vi "XLP80_CAN_VerifyEnums.vi"(8 "err in":errorcluster caption="error") -> (0 "err out":errorcluster caption="error")   [LabVIEW 2021]
uses:
  XLP80_FGlob/1886_FGlob_TDefEnumCANReadItems_Testmode_A.ctl
  XLP80_FGlob/1886_FGlob_TDefEnumCANWriteItems.ctl
  XLP80_Globals/Globals_Settings_XLP80.vi
panel:
  in  "CAN Write Items Testmode_A":T1
  in  "CAN Read Items Testmode_A":T2
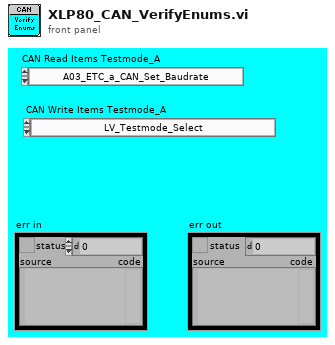
[diagram p1: front panel]
types:
  T1 = typedef "1886_FGlob_TDefEnumCANWriteItems.ctl" = enum16{"LV_Testmode_Select", "LV_A_71_Current_Out_Set", "LV_A_71_Voltage_In_Set", "LV_A_71_Voltage_Out_Set", "LV_H_51_STK_CellVoltages_Enable", "S80_BP_s_Taster_Start_Status"}
  T2 = typedef "1886_FGlob_TDefEnumCANReadItems_Testmode_A.ctl" = enum16{"A03_ETC_a_CAN_Set_Baudrate", "A03_ETC_a_CAN_Set_Broadcast", "A03_ETC_a_CAN_Set_ID_Offset", "A03_ETC_a_CAN_Set_Termination", "A03_ETC_a_CAN_Set_Timeout", "A03_ETC_a_CAN_Set_Timeout_Dur", "A03_ETC_a_Diag_Rq_Select", "A03_ETC_a_Info_Rq_Select", "A03_ETC_a_opCmd1_Error_Ack", "A03_ETC_a_opCmd1_Start_Stop", "A03_ETC_a_opCmd2", "A03_ETC_a_Param_Rq_Select", "A03_ETC_a_SP_In_Press_Enable", "A03_ETC_a_SP_In_Temp_Enable", "A03_ETC_a_SP_Inlet_Pressure", "A03_ETC_a_SP_Inlet_Temperature", "A03_ETC_a_SP_Massflow", "A03_ETC_a_SP_Massflow_Enable", "A03_ETC_a_SP_Out_Press_Enable", "A03_ETC_a_SP_Outlet_Pressure", "A03_ETC_a_Speed_Set", "A03_ETC_s_Converter_Temperature", "A03_ETC_s_Error_Code_1", "A03_ETC_s_Error_Code_2", "A03_ETC_s_HV_In_Voltage", "A03_ETC_s_Information_Code", "A03_ETC_s_LV_In_Voltage", "A03_ETC_s_Output_Power", "A03_ETC_s_Phase_Current", "A03_ETC_s_Phase_Current_Ref", "A03_ETC_s_Phase_Voltage", "A03_ETC_s_PT100_Temperature", "A03_ETC_s_Speed_Actual", "A03_ETC_s_Speed_Reference", "A03_ETC_s_Status1", "A03_ETC_s_Status2", "A03_ETC_s_THC_Temperature", "A03_ETC_s_Warning_Code", "A11_HBV_a_Mode_Set", "A11_HBV_a_Valve_Set", "A11_HBV_s_Mode_Act", "A11_HBV_s_Valve_Act", "A12_SIV_a_Mode_Set", "A12_SIV_a_Valve_Set", "A12_SIV_s_Mode_Act", "A12_SIV_s_Valve_Act", "A13_SOV_a_Mode_Set", "A13_SOV_a_Valve_Set", "A13_SOV_s_Mode_Act", "A13_SOV_s_Valve_Act", "A14_HFM_s_AirMassFlow", "A14_HFM_s_Error_MassFlow", "A14_HFM_s_Error_Pressure", "A14_HFM_s_ErrorCode", "A14_HFM_s_Humidity", "A14_HFM_s_HumidTemperature", "A14_HFM_s_Pressure", "A14_HFM_s_Temperature", "A15_SI_s_Inlet_Pressure", "A16_SI_s_Inlet_Temperature", "A17_SO_s_Outlet_Pressure", "A17_SO_s_Outlet_Temperature", "A22_HSI_s_Humidity", "A23_HSO_s_Humidity", "A56_SO_s_Temperature", "C01_RF_a_FanSpeed", "C01_RF_s_Status", "C02_CP_a_RPM", "C04_DI_s_Temperature", "C06_ET_s_CoolLevelStatus", "C07_BAT_s_BatError_DataValid", "C07_BAT_s_BatError_Intern", "C07_BAT_s_BatError_Temperature", "C07_BAT_s_BatError_Voltage", "C07_BAT_s_Battery_Voltage", "C07_BAT_s_Board_Temperature", "C07_BAT_s_CECUError_Communicat", "C07_BAT_s_CECUError_Current", "C07_BAT_s_CECUError_Intern", "C07_BAT_s_CECUError_Reserved", "C07_BAT_s_CECUError_Service", "C07_BAT_s_CECUError_Supply", "C07_BAT_s_CECUError_Temperature", "C07_BAT_s_CECUError_Voltage", "C07_BAT_s_External_Chrg_Voltage", "C07_BAT_s_External_Load_Voltage", "C07_BAT_s_Max_Cell_Temperature", "C07_BAT_s_Max_Cell_Voltage", "C07_BAT_s_Min_Cell_Temperature", "C07_BAT_s_Min_Cell_Voltage", "C07_BAT_s_PreWarning_Current_H", "C07_BAT_s_PreWarning_SOC_Low", "C07_BAT_s_PreWarning_Temperature", "C07_BAT_s_PreWarning_Voltage_HL", "C07_BAT_s_State", "C07_BAT_s_System_Current", "C08_AMB_s_Humidity_Rel", "C08_AMB_s_Humidity_Spec", "C08_AMB_s_Pressure", "C08_AMB_s_Temperature", "C54_SI_s_Temperature", "C_07_BAT_s_SoC", "C_07_BAT_s_SoH", "E71_DC4880_a_Current_In_Set", "E71_DC4880_a_Current_Out_Set", "E71_DC4880_a_Mode_Control_On", "E71_DC4880_a_Mode_Precharge_On", "E71_DC4880_a_NMT_Function", "E71_DC4880_a_NMT_Node_ID", "E71_DC4880_a_Voltage_In_Set", "E71_DC4880_a_Voltage_Out_Set", "E71_DC4880_s_Current_In_Actual", "E71_DC4880_s_Current_Out_Actual", "E71_DC4880_s_NMT_State", "E71_DC4880_s_State_Control_OK", "E71_DC4880_s_State_Control_On", "E71_DC4880_s_State_Precharge_On", "E71_DC4880_s_Temperature_1_Act", "E71_DC4880_s_Temperature_2_Act", "E71_DC4880_s_Voltage_In_Actual", "E71_DC4880_s_Voltage_Out_Actual", "E72_DC8024_s_Voltage", "E73_DC8012_s_Voltage", "E74_ISO_a_Rq_D_IMC_MANUFACT_IDX", "E74_ISO_a_Rq_D_IMC_MEAN_FACTOR", "E74_ISO_a_Rq_D_IMC_R_ISOERR_THR", "E74_ISO_a_Rq_D_IMC_R_ISOWRN_THR", "E74_ISO_a_Rq_D_IMC_SELFTEST_SCR", "E74_ISO_a_Rq_D_IMC_VERSION_IDX", "E74_ISO_a_Rq_D_VIFC_HV_REL_CHG", "E74_ISO_a_Rq_D_VIFC_HV_RELAIS", "E74_ISO_a_Rq_D_VIFC_LOCK_MODE", "E74_ISO_a_Rq_D_VIFC_LOCK_PWD", "E74_ISO_a_Rq_D_VIFC_MEAS_MODE", "E74_ISO_a_Rq_D_VIFC_RELAIS_STAT", "E74_ISO_a_Rq_D_VIFC_VERSION_IDX", "E74_ISO_s_D_IMC_HV_1", "E74_ISO_s_D_IMC_HV_2", "E74_ISO_s_D_IMC_MANUFACT_DATA", "E74_ISO_s_D_IMC_MANUFACT_INDEX", "E74_ISO_s_D_IMC_MEAN_FACTOR", "E74_ISO_s_D_IMC_R_ISO", "E74_ISO_s_D_IMC_R_ISO_BIAS", "E74_ISO_s_D_IMC_R_ISO_CNT", "E74_ISO_s_D_IMC_R_ISO_ERR_THR1", "E74_ISO_s_D_IMC_R_ISO_ERR_THR2", "E74_ISO_s_D_IMC_R_ISO_WRN_THR1", "E74_ISO_s_D_IMC_R_ISO_WRN_THR2", "E74_ISO_s_D_IMC_SELFTEST_SCR", "E74_ISO_s_D_IMC_STATUS", "E74_ISO_s_D_IMC_STATUS_EXT", "E74_ISO_s_D_IMC_TEST_CNT", "E74_ISO_s_D_IMC_VERSION_Haupt", "E74_ISO_s_D_IMC_VERSION_INDEX", "E74_ISO_s_D_IMC_VERSION_Neben", "E74_ISO_s_D_IMD_ERROR_CODE", "E74_ISO_s_D_IMD_FAILED_CMD", "E74_ISO_s_D_VIFC_HV_RELAIS", "E74_ISO_s_D_VIFC_HV_RELAIS_ACT", "E74_ISO_s_D_VIFC_HV_RELAIS_CHG", "E74_ISO_s_D_VIFC_HV_RELAIS_STAT", "E74_ISO_s_D_VIFC_IMC_ALIVE", "E74_ISO_s_D_VIFC_LOCK_MODE", "E74_ISO_s_D_VIFC_MEASURE_MODE", "E74_ISO_s_D_VIFC_STATUS", "E74_ISO_s_D_VIFC_VERSION_Haupt", "E74_ISO_s_D_VIFC_VERSION_INDEX", "E74_ISO_s_D_VIFC_VERSION_Neben", "E74_ISO_s_IMC_R_ISO", "E74_ISO_s_IMC_STATUS_ErrChassis", "E74_ISO_s_IMC_STATUS_Isofehler", "E74_ISO_s_IMC_STATUS_Isowarnung", "E74_ISO_s_IMC_STATUS_Kalib", "E74_ISO_s_IMC_STATUS_Selbsttest", "E74_ISO_s_IMC_STATUS_Syststoer", "E74_ISO_s_Rq_D_IMC_MEAN_FACTOR", "E74_ISO_s_VIFC_STATUS_IMC_Alive", "E74_ISO_s_VIFC_STATUS_IMC_St_OA", "E74_ISO_s_VIFC_STATUS_IMC_St_PC", "E74_ISO_s_VIFC_STATUS_IsoAlt", "E74_ISO_s_VIFC_STATUS_Isomess", "E74_ISO_s_VIFC_STATUS_Stoer_IMC", "E74_ISO_s_VIFC_STATUS_VIFC_Cmd", "E75_HVP_a_Relais_Set", "E76_HVM_a_Relais_Set", "E95_DC2405_s_Voltage", "H31_OTV_a_Valve_Set", "H31_OTV_s_Pressure", "H31_OTV_s_Temperature", "H36_GHU_s_Pressure_1", "H37_GHU_s_Temperature_1", "H38_HSV_a_Valve_Set", "H40_GHU_s_Pressure_2", "H41_GHU_s_Temperature_2", "H42_HRB_a_FCCU_CRC", "H42_HRB_a_FCCU_Heating_Rq", "H42_HRB_a_FCCU_Spd_Rq", "H42_HRB_a_FCCU_SQC", "H42_HRB_s_ARB_Batt_Vltg_Err", "H42_HRB_s_ARB_Batt_Voltage", "H42_HRB_s_ARB_Blocked_Err", "H42_HRB_s_ARB_BrdgDrv_Err", "H42_HRB_s_ARB_E2E_Err", "H42_HRB_s_ARB_ECU_P_out", "H42_HRB_s_ARB_ECU_Temp", "H42_HRB_s_ARB_ECU_Temp_DrCnd", "H42_HRB_s_ARB_ECU_Temp_Err", "H42_HRB_s_ARB_ErrCRC", "H42_HRB_s_ARB_ErrSQC", "H42_HRB_s_ARB_I_D_Curr", "H42_HRB_s_ARB_I_Q_Curr", "H42_HRB_s_ARB_Init_Err", "H42_HRB_s_ARB_Mtr_Temp", "H42_HRB_s_ARB_Mtr_Temp_DrCnd", "H42_HRB_s_ARB_Mtr_Temp_Err", "H42_HRB_s_ARB_MtrNTCFlr_DrCnd", "H42_HRB_s_ARB_ShortToBat_Err", "H42_HRB_s_ARB_ShortToGround_Err", "H42_HRB_s_ARB_Spd", "H42_HRB_s_ARB_SpdDiff_DrCnd", "H42_HRB_s_ARB_SpdLimitRq_Err", "H42_HRB_s_ARB_SysState", "H42_HRB_s_ARB_Torque", "H42_HRB_s_ARB_U_D_Volt", "H42_HRB_s_ARB_U_Q_Volt", "H42_HRB_s_BrdgDrv_VCC_UV_Err", "H43_HDV_a_Dosing_Valve_Set", "H45_WT_s_WaterLevelStatus", "H46_HRBo_a_Drain_Valve_Set", "H51_STK_a_AmountOfModules_1002", "H51_STK_a_CAN_TerminatRes_1002", "H51_STK_a_CellsPerModule_1002", "H51_STK_a_CellVoltage_1001", "H51_STK_a_Command_1004", "H51_STK_a_CoreData_1001", "H51_STK_a_CoreData_Freq_1002", "H51_STK_a_DataLength_1001", "H51_STK_a_DataLength_1002", "H51_STK_a_DataLength_1003", "H51_STK_a_DataLength_1004", "H51_STK_a_DataLength_1006", "H51_STK_a_DataLength_100B", "H51_STK_a_DateTime_1002", "H51_STK_a_Diff_MaxMin_limit_1002", "H51_STK_a_FCCUResponse_1006", "H51_STK_a_Firmware_1001", "H51_STK_a_ID_1003", "H51_STK_a_ID_1004", "H51_STK_a_ID_H_1001", "H51_STK_a_ID_H_1002", "H51_STK_a_ID_H_100B", "H51_STK_a_ID_L_100B", "H51_STK_a_Logdata_1001", "H51_STK_a_Lower_Limit2_1002", "H51_STK_a_MasterNo_1002", "H51_STK_a_Modul_100B", "H51_STK_a_Monitoring_Flag_1003", "H51_STK_a_PosAtStack_1002", "H51_STK_a_StackSize_1002", "H51_STK_a_Temperature_1002", "H51_STK_a_Upper_Limit1_1002", "H51_STK_a_UpperLimit2_1002", "H51_STK_s_Amount_Slave_Modu_2000", "H51_STK_s_AmountofContactFailure", "H51_STK_s_AmountOfFrames_2002", "H51_STK_s_AmountOfFrames_2003", "H51_STK_s_AmountOfFrames_2005", "H51_STK_s_AmountOfFrames_2006", "H51_STK_s_AmountOfFrames_2011", "H51_STK_s_AverageTemp_2004", "H51_STK_s_CellContactNr10_2006", "H51_STK_s_CellContactNr11_2006", "H51_STK_s_CellContactNr12_2006", "H51_STK_s_CellContactNr13_2006", "H51_STK_s_CellContactNr14_2006", "H51_STK_s_CellContactNr15_2006", "H51_STK_s_CellContactNr16_2006", "H51_STK_s_CellContactNr17_2006", "H51_STK_s_CellContactNr18_2006", "H51_STK_s_CellContactNr19_2006", "H51_STK_s_CellContactNr1_2006", "H51_STK_s_CellContactNr20_2006", "H51_STK_s_CellContactNr21_2006", "H51_STK_s_CellContactNr22_2006", "H51_STK_s_CellContactNr23_2006", "H51_STK_s_CellContactNr24_2006", "H51_STK_s_CellContactNr25_2006", "H51_STK_s_CellContactNr26_2006", "H51_STK_s_CellContactNr27_2006", "H51_STK_s_CellContactNr28_2006", "H51_STK_s_CellContactNr29_2006", "H51_STK_s_CellContactNr2_2006", "H51_STK_s_CellContactNr30_2006", "H51_STK_s_CellContactNr31_2006", "H51_STK_s_CellContactNr32_2006", "H51_STK_s_CellContactNr33_2006", "H51_STK_s_CellContactNr34_2006", "H51_STK_s_CellContactNr35_2006", "H51_STK_s_CellContactNr36_2006", "H51_STK_s_CellContactNr37_2006", "H51_STK_s_CellContactNr38_2006", "H51_STK_s_CellContactNr39_2006", "H51_STK_s_CellContactNr3_2006", "H51_STK_s_CellContactNr40_2006", "H51_STK_s_CellContactNr41_2006", "H51_STK_s_CellContactNr42_2006", "H51_STK_s_CellContactNr43_2006", "H51_STK_s_CellContactNr44_2006", "H51_STK_s_CellContactNr45_2006", "H51_STK_s_CellContactNr46_2006", "H51_STK_s_CellContactNr47_2006", "H51_STK_s_CellContactNr48_2006", "H51_STK_s_CellContactNr49_2006", "H51_STK_s_CellContactNr4_2006", "H51_STK_s_CellContactNr50_2006", "H51_STK_s_CellContactNr51_2006", "H51_STK_s_CellContactNr52_2006", "H51_STK_s_CellContactNr53_2006", "H51_STK_s_CellContactNr54_2006", "H51_STK_s_CellContactNr55_2006", "H51_STK_s_CellContactNr56_2006", "H51_STK_s_CellContactNr57_2006", "H51_STK_s_CellContactNr58_2006", "H51_STK_s_CellContactNr59_2006", "H51_STK_s_CellContactNr5_2006", "H51_STK_s_CellContactNr60_2006", "H51_STK_s_CellContactNr61_2006", "H51_STK_s_CellContactNr62_2006", "H51_STK_s_CellContactNr63_2006", "H51_STK_s_CellContactNr64_2006", "H51_STK_s_CellContactNr65_2006", "H51_STK_s_CellContactNr66_2006", "H51_STK_s_CellContactNr67_2006", "H51_STK_s_CellContactNr68_2006", "H51_STK_s_CellContactNr69_2006", "H51_STK_s_CellContactNr6_2006", "H51_STK_s_CellContactNr70_2006", "H51_STK_s_CellContactNr71_2006", "H51_STK_s_CellContactNr7_2006", "H51_STK_s_CellContactNr8_2006", "H51_STK_s_CellContactNr9_2006", "H51_STK_s_CellNo_2ndlow_2003", "H51_STK_s_CellNo_highest_2003", "H51_STK_s_CellNo_lowest_2003", "H51_STK_s_CellVolt_001_2005", "H51_STK_s_CellVolt_002_2005", "H51_STK_s_CellVolt_003_2005", "H51_STK_s_CellVolt_004_2005", "H51_STK_s_CellVolt_005_2005", "H51_STK_s_CellVolt_006_2005", "H51_STK_s_CellVolt_007_2005", "H51_STK_s_CellVolt_008_2005", "H51_STK_s_CellVolt_009_2005", "H51_STK_s_CellVolt_010_2005", "H51_STK_s_CellVolt_011_2005", "H51_STK_s_CellVolt_012_2005", "H51_STK_s_CellVolt_013_2005", "H51_STK_s_CellVolt_014_2005", "H51_STK_s_CellVolt_015_2005", "H51_STK_s_CellVolt_016_2005", "H51_STK_s_CellVolt_017_2005", "H51_STK_s_CellVolt_018_2005", "H51_STK_s_CellVolt_019_2005", "H51_STK_s_CellVolt_020_2005", "H51_STK_s_CellVolt_021_2005", "H51_STK_s_CellVolt_022_2005", "H51_STK_s_CellVolt_023_2005", "H51_STK_s_CellVolt_024_2005", "H51_STK_s_CellVolt_025_2005", "H51_STK_s_CellVolt_026_2005", "H51_STK_s_CellVolt_027_2005", "H51_STK_s_CellVolt_028_2005", "H51_STK_s_CellVolt_029_2005", "H51_STK_s_CellVolt_030_2005", "H51_STK_s_CellVolt_031_2005", "H51_STK_s_CellVolt_032_2005", "H51_STK_s_CellVolt_033_2005", "H51_STK_s_CellVolt_034_2005", "H51_STK_s_CellVolt_035_2005", "H51_STK_s_CellVolt_036_2005", "H51_STK_s_CellVolt_037_2005", "H51_STK_s_CellVolt_038_2005", "H51_STK_s_CellVolt_039_2005", "H51_STK_s_CellVolt_040_2005", "H51_STK_s_CellVolt_041_2005", "H51_STK_s_CellVolt_042_2005", "H51_STK_s_CellVolt_043_2005", "H51_STK_s_CellVolt_044_2005", "H51_STK_s_CellVolt_045_2005", "H51_STK_s_CellVolt_046_2005", "H51_STK_s_CellVolt_047_2005", "H51_STK_s_CellVolt_048_2005", "H51_STK_s_CellVolt_049_2005", "H51_STK_s_CellVolt_050_2005", "H51_STK_s_CellVolt_051_2005", "H51_STK_s_CellVolt_052_2005", "H51_STK_s_CellVolt_053_2005", "H51_STK_s_CellVolt_054_2005", "H51_STK_s_CellVolt_055_2005", "H51_STK_s_CellVolt_056_2005", "H51_STK_s_CellVolt_057_2005", "H51_STK_s_CellVolt_058_2005", "H51_STK_s_CellVolt_059_2005", "H51_STK_s_CellVolt_060_2005", "H51_STK_s_CellVolt_061_2005", "H51_STK_s_CellVolt_062_2005", "H51_STK_s_CellVolt_063_2005", "H51_STK_s_CellVolt_064_2005", "H51_STK_s_CellVolt_065_2005", "H51_STK_s_CellVolt_066_2005", "H51_STK_s_CellVolt_067_2005", "H51_STK_s_CellVolt_068_2005", "H51_STK_s_CellVolt_069_2005", "H51_STK_s_CellVolt_070_2005", "H51_STK_s_CellVolt_071_2005", "H51_STK_s_CellVolt_2ndlow_2003", "H51_STK_s_CellVolt_follow_2ndlow", "H51_STK_s_CellVolt_follow_lowest", "H51_STK_s_CellVolt_highest_2003", "H51_STK_s_CellVolt_lowest_2003", "H51_STK_s_CellVolt_prev_2ndlow", "H51_STK_s_CellVolt_prev_lowest", "H51_STK_s_CellVoltage_ui16H_2004", "H51_STK_s_CellVoltage_ui16L_2004", "H51_STK_s_Contact_Cell_10_2010", "H51_STK_s_Contact_Cell_11_2010", "H51_STK_s_Contact_Cell_12_2010", "H51_STK_s_Contact_Cell_13_2010", "H51_STK_s_Contact_Cell_14_2010", "H51_STK_s_Contact_Cell_15_2010", "H51_STK_s_Contact_Cell_16_2010", "H51_STK_s_Contact_Cell_17_2010", "H51_STK_s_Contact_Cell_18_2010", "H51_STK_s_Contact_Cell_19_2010", "H51_STK_s_Contact_Cell_1_2010", "H51_STK_s_Contact_Cell_20_2010", "H51_STK_s_Contact_Cell_21_2010", "H51_STK_s_Contact_Cell_22_2010", "H51_STK_s_Contact_Cell_23_2010", "H51_STK_s_Contact_Cell_24_2010", "H51_STK_s_Contact_Cell_25_2010", "H51_STK_s_Contact_Cell_26_2010", "H51_STK_s_Contact_Cell_27_2010", "H51_STK_s_Contact_Cell_28_2010", "H51_STK_s_Contact_Cell_29_2010", "H51_STK_s_Contact_Cell_2_2010", "H51_STK_s_Contact_Cell_30_2010", "H51_STK_s_Contact_Cell_31_2010", "H51_STK_s_Contact_Cell_32_2010", "H51_STK_s_Contact_Cell_33_2010", "H51_STK_s_Contact_Cell_34_2010", "H51_STK_s_Contact_Cell_35_2010", "H51_STK_s_Contact_Cell_36_2010", "H51_STK_s_Contact_Cell_37_2010", "H51_STK_s_Contact_Cell_38_2010", "H51_STK_s_Contact_Cell_39_2010", "H51_STK_s_Contact_Cell_3_2010", "H51_STK_s_Contact_Cell_40_2010", "H51_STK_s_Contact_Cell_41_2010", "H51_STK_s_Contact_Cell_42_2010", "H51_STK_s_Contact_Cell_43_2010", "H51_STK_s_Contact_Cell_44_2010", "H51_STK_s_Contact_Cell_45_2010", "H51_STK_s_Contact_Cell_46_2010", "H51_STK_s_Contact_Cell_47_2010", "H51_STK_s_Contact_Cell_48_2010", "H51_STK_s_Contact_Cell_49_2010", "H51_STK_s_Contact_Cell_4_2010", "H51_STK_s_Contact_Cell_50_2010", "H51_STK_s_Contact_Cell_51_2010", "H51_STK_s_Contact_Cell_52_2010", "H51_STK_s_Contact_Cell_53_2010", "H51_STK_s_Contact_Cell_54_2010", "H51_STK_s_Contact_Cell_55_2010", "H51_STK_s_Contact_Cell_56_2010", "H51_STK_s_Contact_Cell_57_2010", "H51_STK_s_Contact_Cell_58_2010", "H51_STK_s_Contact_Cell_59_2010", "H51_STK_s_Contact_Cell_5_2010", "H51_STK_s_Contact_Cell_60_2010", "H51_STK_s_Contact_Cell_61_2010", "H51_STK_s_Contact_Cell_62_2010", "H51_STK_s_Contact_Cell_63_2010", "H51_STK_s_Contact_Cell_64_2010", "H51_STK_s_Contact_Cell_65_2010", "H51_STK_s_Contact_Cell_66_2010", "H51_STK_s_Contact_Cell_67_2010", "H51_STK_s_Contact_Cell_68_2010", "H51_STK_s_Contact_Cell_69_2010", "H51_STK_s_Contact_Cell_6_2010", "H51_STK_s_Contact_Cell_70_2010", "H51_STK_s_Contact_Cell_71_2010", "H51_STK_s_Contact_Cell_7_2010", "H51_STK_s_Contact_Cell_8_2010", "H51_STK_s_Contact_Cell_9_2010", "H51_STK_s_CVM_Firmw_Master_2002", "H51_STK_s_CVM_Firmw_Slave10_2002", "H51_STK_s_CVM_Firmw_Slave11_2002", "H51_STK_s_CVM_Firmw_Slave12_2002", "H51_STK_s_CVM_Firmw_Slave13_2002", "H51_STK_s_CVM_Firmw_Slave14_2002", "H51_STK_s_CVM_Firmw_Slave15_2002", "H51_STK_s_CVM_Firmw_Slave16_2002", "H51_STK_s_CVM_Firmw_Slave17_2002", "H51_STK_s_CVM_Firmw_Slave18_2002", "H51_STK_s_CVM_Firmw_Slave19_2002", "H51_STK_s_CVM_Firmw_Slave1_2002", "H51_STK_s_CVM_Firmw_Slave20_2002", "H51_STK_s_CVM_Firmw_Slave21_2002", "H51_STK_s_CVM_Firmw_Slave22_2002", "H51_STK_s_CVM_Firmw_Slave23_2002", "H51_STK_s_CVM_Firmw_Slave24_2002", "H51_STK_s_CVM_Firmw_Slave2_2002", "H51_STK_s_CVM_Firmw_Slave3_2002", "H51_STK_s_CVM_Firmw_Slave4_2002", "H51_STK_s_CVM_Firmw_Slave5_2002", "H51_STK_s_CVM_Firmw_Slave6_2002", "H51_STK_s_CVM_Firmw_Slave7_2002", "H51_STK_s_CVM_Firmw_Slave8_2002", "H51_STK_s_CVM_Firmw_Slave9_2002", "H51_STK_s_CVMResponse_200F", "H51_STK_s_DataLength_2000", "H51_STK_s_Datalength_2001", "H51_STK_s_Datalength_2004", "H51_STK_s_DataLength_200F", "H51_STK_s_DataLength_CVM_2010", "H51_STK_s_EventNo_2004", "H51_STK_s_ID_2001", "H51_STK_s_ID_H_2000", "H51_STK_s_ID_H_2002", "H51_STK_s_ID_H_200F", "H51_STK_s_ID_L_2000", "H51_STK_s_ID_L_2002", "H51_STK_s_ID_L_200F", "H51_STK_s_MasterBMS1REF1_2011", "H51_STK_s_MasterBMS1REF2_2011", "H51_STK_s_MasterBMS2REF1_2011", "H51_STK_s_MasterBMS2REF2_2011", "H51_STK_s_ModulHighestTemp_2003", "H51_STK_s_ModulNr_HighestTemp", "H51_STK_s_RequestBit_2001", "H51_STK_s_Slave10BMS1REF1_2011", "H51_STK_s_Slave10BMS1REF2_2011", "H51_STK_s_Slave10BMS2REF1_2011", "H51_STK_s_Slave10BMS2REF2_2011", "H51_STK_s_Slave11BMS1REF1_2011", "H51_STK_s_Slave11BMS1REF2_2011", "H51_STK_s_Slave11BMS2REF1_2011", "H51_STK_s_Slave11BMS2REF2_2011", "H51_STK_s_Slave12BMS1REF1_2011", "H51_STK_s_Slave12BMS1REF2_2011", "H51_STK_s_Slave12BMS2REF1_2011", "H51_STK_s_Slave12BMS2REF2_2011", "H51_STK_s_Slave13BMS1REF1_2011", "H51_STK_s_Slave13BMS1REF2_2011", "H51_STK_s_Slave13BMS2REF1_2011", "H51_STK_s_Slave13BMS2REF2_2011", "H51_STK_s_Slave14BMS1REF1_2011", "H51_STK_s_Slave14BMS1REF2_2011", "H51_STK_s_Slave14BMS2REF1_2011", "H51_STK_s_Slave14BMS2REF2_2011", "H51_STK_s_Slave15BMS1REF1_2011", "H51_STK_s_Slave15BMS1REF2_2011", "H51_STK_s_Slave15BMS2REF1_2011", "H51_STK_s_Slave15BMS2REF2_2011", "H51_STK_s_Slave16BMS1REF1_2011", "H51_STK_s_Slave16BMS1REF2_2011", "H51_STK_s_Slave16BMS2REF1_2011", "H51_STK_s_Slave16BMS2REF2_2011", "H51_STK_s_Slave17BMS1REF1_2011", "H51_STK_s_Slave17BMS1REF2_2011", "H51_STK_s_Slave17BMS2REF1_2011", "H51_STK_s_Slave17BMS2REF2_2011", "H51_STK_s_Slave18BMS1REF1_2011", "H51_STK_s_Slave18BMS1REF2_2011", "H51_STK_s_Slave18BMS2REF1_2011", "H51_STK_s_Slave18BMS2REF2_2011", "H51_STK_s_Slave19BMS1REF1_2011", "H51_STK_s_Slave19BMS1REF2_2011", "H51_STK_s_Slave19BMS2REF1_2011", "H51_STK_s_Slave19BMS2REF2_2011", "H51_STK_s_Slave1BMS1REF1_2011", "H51_STK_s_Slave1BMS1REF2_2011", "H51_STK_s_Slave1BMS2REF1_2011", "H51_STK_s_Slave1BMS2REF2_2011", "H51_STK_s_Slave20BMS1REF1_2011", "H51_STK_s_Slave20BMS1REF2_2011", "H51_STK_s_Slave20BMS2REF1_2011", "H51_STK_s_Slave20BMS2REF2_2011", "H51_STK_s_Slave21BMS1REF1_2011", "H51_STK_s_Slave21BMS1REF2_2011", "H51_STK_s_Slave21BMS2REF1_2011", "H51_STK_s_Slave21BMS2REF2_2011", "H51_STK_s_Slave22BMS1REF1_2011", "H51_STK_s_Slave22BMS1REF2_2011", "H51_STK_s_Slave22BMS2REF1_2011", "H51_STK_s_Slave22BMS2REF2_2011", "H51_STK_s_Slave23BMS1REF1_2011", "H51_STK_s_Slave23BMS1REF2_2011", "H51_STK_s_Slave23BMS2REF1_2011", "H51_STK_s_Slave23BMS2REF2_2011", "H51_STK_s_Slave24BMS1REF1_2011", "H51_STK_s_Slave24BMS1REF2_2011", "H51_STK_s_Slave24BMS2REF1_2011", "H51_STK_s_Slave24BMS2REF2_2011", "H51_STK_s_Slave25BMS1REF1_2011", "H51_STK_s_Slave25BMS1REF2_2011", "H51_STK_s_Slave25BMS2REF1_2011", "H51_STK_s_Slave25BMS2REF2_2011", "H51_STK_s_Slave2BMS1REF1_2011", "H51_STK_s_Slave2BMS1REF2_2011", "H51_STK_s_Slave2BMS2REF1_2011", "H51_STK_s_Slave2BMS2REF2_2011", "H51_STK_s_Slave3BMS1REF1_2011", "H51_STK_s_Slave3BMS1REF2_2011", "H51_STK_s_Slave3BMS2REF1_2011", "H51_STK_s_Slave3BMS2REF2_2011", "H51_STK_s_Slave4BMS1REF1_2011", "H51_STK_s_Slave4BMS1REF2_2011", "H51_STK_s_Slave4BMS2REF1_2011", "H51_STK_s_Slave4BMS2REF2_2011", "H51_STK_s_Slave5BMS1REF1_2011", "H51_STK_s_Slave5BMS1REF2_2011", "H51_STK_s_Slave5BMS2REF1_2011", "H51_STK_s_Slave5BMS2REF2_2011", "H51_STK_s_Slave6BMS1REF1_2011", "H51_STK_s_Slave6BMS1REF2_2011", "H51_STK_s_Slave6BMS2REF1_2011", "H51_STK_s_Slave6BMS2REF2_2011", "H51_STK_s_Slave7BMS1REF1_2011", "H51_STK_s_Slave7BMS1REF2_2011", "H51_STK_s_Slave7BMS2REF1_2011", "H51_STK_s_Slave7BMS2REF2_2011", "H51_STK_s_Slave8BMS1REF1_2011", "H51_STK_s_Slave8BMS1REF2_2011", "H51_STK_s_Slave8BMS2REF1_2011", "H51_STK_s_Slave8BMS2REF2_2011", "H51_STK_s_Slave9BMS1REF1_2011", "H51_STK_s_Slave9BMS1REF2_2011", "H51_STK_s_Slave9BMS2REF1_2011", "H51_STK_s_Slave9BMS2REF2_2011", "H51_STK_s_Stat_CVM_Mastermo_2000", "H51_STK_s_TotalVoltage_2003", "H51_STK_s_Watchdog_2000", "H51_STK_s_ZellNo_2004", "H52_DV_a_Drain_Valve_Stack_Set", "H53_PV_a_Purge_Valve_Stack_Set", "H55_SI_s_Stack_Inlet_Pressure", "H62_HLD_s_1_CRC8", "H62_HLD_s_1_CycleCounter", "H62_HLD_s_1_Engineer_Info_1", "H62_HLD_s_1_Engineer_Info_2", "H62_HLD_s_1_Engineer_Info_3", "H62_HLD_s_1_Engineer_Info_4", "H62_HLD_s_1_H2_Concentration", "H62_HLD_s_1_HW_Type", "H62_HLD_s_1_HW_Version", "H62_HLD_s_1_Sensor_ErrorCode", "H62_HLD_s_1_SensorID", "H62_HLD_s_1_SW_Version_Main", "H62_HLD_s_1_SW_Version_Sub", "H62_HLD_s_2_CRC8", "H62_HLD_s_2_CycleCounter", "H62_HLD_s_2_Engineer_Info_1", "H62_HLD_s_2_Engineer_Info_2", "H62_HLD_s_2_Engineer_Info_3", "H62_HLD_s_2_Engineer_Info_4", "H62_HLD_s_2_H2_Concentration", "H62_HLD_s_2_HW_Type", "H62_HLD_s_2_HW_Version", "H62_HLD_s_2_Sensor_ErrorCode", "H62_HLD_s_2_SensorID", "H62_HLD_s_2_SW_Version_Main", "H62_HLD_s_2_SW_Version_Sub", "H63_HLD_s_1_CRC8", "H63_HLD_s_1_CycleCounter", "H63_HLD_s_1_Engineer_Info_1", "H63_HLD_s_1_Engineer_Info_2", "H63_HLD_s_1_Engineer_Info_3", "H63_HLD_s_1_Engineer_Info_4", "H63_HLD_s_1_H2_Concentration", "H63_HLD_s_1_HW_Type", "H63_HLD_s_1_HW_Version", "H63_HLD_s_1_Sensor_ErrorCode", "H63_HLD_s_1_SensorID", "H63_HLD_s_1_SW_Version_Main", "H63_HLD_s_1_SW_Version_Sub", "H63_HLD_s_2_CRC8", "H63_HLD_s_2_CycleCounter", "H63_HLD_s_2_Engineer_Info_1", "H63_HLD_s_2_Engineer_Info_2", "H63_HLD_s_2_Engineer_Info_3", "H63_HLD_s_2_Engineer_Info_4", "H63_HLD_s_2_H2_Concentration", "H63_HLD_s_2_HW_Type", "H63_HLD_s_2_HW_Version", "H63_HLD_s_2_Sensor_ErrorCode", "H63_HLD_s_2_SensorID", "H63_HLD_s_2_SW_Version_Main", "H63_HLD_s_2_SW_Version_Sub", "LV_Testmode_Select", "S80_BP_a_Bat_Control_LED_On", "S80_BP_a_Beep_On", "S80_BP_a_Distance_Horizontal", "S80_BP_a_Distance_Vertical", "S80_BP_a_FuelLevel_Display", "S80_BP_a_H2_Water_Ctrl_LED_On", "S80_BP_a_Leakage_LED_On", "S80_BP_a_Service_LED_On", "S80_BP_a_Taster_Start_LED_On", "S80_BP_a_Taster_Stop_LED_On", "S80_BP_a_WiFi_Status", "S80_BP_s_Taster_Start_Status", "S80_BP_s_Taster_Stop_Status", "S83_DCO_s_Wifi_Status", "S83_en_p_cldn_amblimit_temp", "S83_en_p_cldn_amblimitoff_temp", "S83_en_p_cldn_cp_spd", "S83_en_p_cldn_rf_spd", "S83_en_p_cldn_rf_time", "S83_en_p_cldn_soclimit", "S83_en_p_cldn_time2off", "S83_en_p_cvm_diff_maxmin_lim", "S83_en_p_cvm_frequency", "S83_en_p_cvm_low_lim2", "S83_en_p_cvm_temperature", "S83_en_p_cvm_up_lim1", "S83_en_p_cvm_up_lim2", "S83_en_p_fca_etc_preset_gradient", "S83_en_p_fcdu_stk_curr_ramp_time", "S83_en_p_fcsd_etc_initrng_spd", "S83_en_p_fcsd_h2end_press", "S83_en_p_fcsd_hrbstp_spd", "S83_en_p_fcsu_bpv_opncls_time", "S83_en_p_fcsu_dcdc_currrampgrad", "S83_en_p_fcsu_dcdc_maxwrmup_curr", "S83_en_p_fcsu_dcdc_optime", "S83_en_p_fcsu_dcdc_preoptime", "S83_en_p_fcsu_etc_initspd", "S83_en_p_fcsu_ghu_strtpress1", "S83_en_p_fcsu_ghu_strtpress2", "S83_en_p_fcsu_h2_initpress", "S83_en_p_fcsu_h2_strtpress", "S83_en_p_fcsu_hrb_strtspd", "S83_en_p_fcsu_initmincellvolt", "S83_en_p_fcsu_mincellvolt_time", "S83_en_p_fcsu_pvrmp_incrclstime", "S83_en_p_fcsu_pvrmp_opntime", "S83_en_p_fcsu_pvrmp_strtclstime", "S83_en_p_fcsu_stk_deltamedlow_v", "S83_en_p_fcsu_stk_lowcellvolt", "S83_en_p_fcsu_stk_normopset_temp", "S83_en_p_hmi_bat_soc_limit_low", "S83_en_p_hmi_bat_soc_limit_ok", "S83_en_p_hmi_h2_leak_amb_ppm", "S83_en_p_hmi_h2_leak_exh_ppm", "S83_en_p_hmi_h2_leak_exh_s", "S83_en_p_hmi_h2tanklvl_displ", "S83_en_p_hmi_h2tanklvl_presslim", "S83_en_p_hmi_h2tanklvl_scale0", "S83_en_p_hmi_h2tanklvl_scale1", "S83_en_p_hrbo_a_valve_async_fact", "S83_en_p_hrbo_a_valve_i_fact", "S83_en_p_hrbo_a_valve_ot_fact", "S83_en_p_p_minucell_range1_time", "S83_en_p_p_minucell_range1_volt", "S83_en_p_p_minucell_range2_time", "S83_en_p_p_minucell_range2_volt", "S83_en_p_pc_uirangecell_time", "S83_en_p_pc_uirangecell_volt", "S83_en_p_power_out_fc_high", "S83_en_p_power_out_fc_low", "S83_en_p_rfc_hghvent_fanspd", "S83_en_p_rfc_nrmopbaseval_fanspd", "S83_en_p_rfc_srtstpvent_fanspd", "S83_en_p_soc_limit_fc_high", "S83_en_p_soc_limit_fc_low", "S83_en_p_soc_limit_fc_off", "S83_en_p_spdn_batlimit_curr", "S83_en_p_spdn_batlimit_time", "S83_en_p_tc_clpmpspd_idx0", "S83_en_p_tc_clpmpspd_idx1", "S83_en_p_tc_clpmpspd_idx2", "S83_en_P_TC_GHU_maxlowpress", "S83_en_P_TC_GHU_maxmidpress", "S83_en_P_TC_OTV_maxtankpress", "S83_en_p_wtlc_soc_lvl_perc", "S83_en_p_wtlc_soc_time2off_sec", "S83_P_CLDN_AMBlimit_Temp", "S83_P_CLDN_AMBlimitOff_Temp", "S83_P_CLDN_CP_Spd", "S83_P_CLDN_RF_Spd", "S83_P_CLDN_RF_Time", "S83_P_CLDN_SOClimit", "S83_P_CLDN_time2off", "S83_P_CVM_Diff_MaxMin_Lim", "S83_P_CVM_Frequency", "S83_P_CVM_Low_Lim2", "S83_P_CVM_Temperature", "S83_P_CVM_Up_Lim1", "S83_P_CVM_Up_Lim2", "S83_P_FCA_ETC_Preset_Gradient", "S83_P_FCA_Press_D_Ctrl", "S83_P_FCA_Press_I_Ctrl", "S83_P_FCA_Press_P_Ctrl", "S83_P_FCDU_STK_Curr_Ramp_Time", "S83_P_FCH_Press_D_Ctrl", "S83_P_FCH_Press_I_Ctrl", "S83_P_FCH_Press_P_Ctrl", "S83_P_FCSD_H2end_Press", "S83_P_FCSD_HRBstp_Spd", "S83_P_FCSU_DCDC_CurrRampGrad", "S83_P_FCSU_DCDC_OpTime", "S83_P_FCSU_DCDC_PreOpTime", "S83_P_FCSU_ETC_InitSpd", "S83_P_FCSU_GHU_StrtPress1", "S83_P_FCSU_GHU_StrtPress2", "S83_P_FCSU_H2_InitPress", "S83_P_FCSU_H2_Press_I_Ctrl", "S83_P_FCSU_H2_Press_P_Ctrl", "S83_P_FCSU_H2_StrtPress", "S83_P_FCSU_HRB_StrtSpd", "S83_P_FCSU_InitMinCellVolt", "S83_P_FCSU_MinCellVolt_Time", "S83_P_FCSU_PVrmp_IncrClsTime", "S83_P_FCSU_PVrmp_IniOpnTime", "S83_P_FCSU_PVrmp_StrtClsTime", "S83_P_FCSU_STK_DeltaMedLow_V", "S83_P_FCSU_STK_LowCellVolt", "S83_P_FCSU_STK_NormOpSet_Temp", "S83_P_HMI_BAT_SOC_Limit_low", "S83_P_HMI_BAT_SOC_Limit_ok", "S83_P_HMI_H2_leak_amb_ppm", "S83_P_HMI_H2_leak_exh_ppm", "S83_P_HMI_H2_leak_exh_s", "S83_P_HMI_H2TankLvl_Displ", "S83_P_HMI_H2TankLvl_PressLim", "S83_P_HMI_H2TankLvl_Scale0", "S83_P_HMI_H2TankLvl_Scale1", "S83_P_HRBo_a_Valve_Async_fact", "S83_P_HRBo_a_Valve_I_fact", "S83_P_HRBo_a_Valve_OT_fact", "S83_P_PC_MinUCell_range1_Time", "S83_P_PC_MinUCell_range1_Volt", "S83_P_PC_MinUCell_range2_Time", "S83_P_PC_MinUCell_range2_Volt", "S83_P_PC_UIrangeCell_Time", "S83_P_PC_UIrangeCell_Volt", "S83_P_Power_Out_FC_High", "S83_P_Power_Out_FC_Low", "S83_P_RFC_HghVent_FanSpd", "S83_P_RFC_NrmOpBaseVal_FanSpd", "S83_P_RFC_SrtStpVent_FanSpd", "S83_P_SOC_Limit_FC_High", "S83_P_SOC_Limit_FC_Low", "S83_P_SOC_Limit_FC_Off", "S83_P_SPDN_BATlimit_Curr", "S83_P_TC_ClPmpSpd_Amp0", "S83_P_TC_ClPmpSpd_Amp1", "S83_P_TC_ClPmpSpd_Amp2", "S83_P_TC_ClPmpSpd_perc0", "S83_P_TC_ClPmpSpd_perc1", "S83_P_TC_ClPmpSpd_perc2", "S83_P_TC_GHU_MaxLowPress", "S83_P_TC_GHU_MaxMidPress", "S83_P_TC_OTV_MaxTankPress", "S83_P_TC_StkIntT_P_Crtl_FanSpd", "S83_P_WTLC_SOC_Lvl", "S83_P_WTLC_SOC_time2off", "S91_en_p_fca_etc_preset_gradient", "S91_en_p_fcdu_stk_curr_ramp_time", "S91_LV_Testmode", "S91_P_CLDN_AMBlimit_Temp", "S91_P_CLDN_AMBlimitOff_Temp", "S91_P_CLDN_CP_Spd", "S91_P_CLDN_RF_Spd", "S91_P_CLDN_RF_Time", "S91_P_CLDN_SOClimit", "S91_P_CLDN_time2off", "S91_P_CVM_Diff_MaxMin_Lim", "S91_P_CVM_Frequency", "S91_P_CVM_Low_Lim2", "S91_P_CVM_Temperature", "S91_P_CVM_Up_Lim1", "S91_P_CVM_Up_Lim2", "S91_P_FCA_ETC_Preset_Gradient", "S91_P_FCA_Press_D_Ctrl", "S91_P_FCA_Press_I_Ctrl", "S91_P_FCA_Press_P_Ctrl", "S91_P_FCDU_STK_Curr_Ramp_Time", "S91_P_FCH_Press_D_Ctrl", "S91_P_FCH_Press_I_Ctrl", "S91_P_FCH_Press_P_Ctrl", "S91_P_FCSD_ETC_InitRng_Spd", "S91_P_FCSD_H2end_Press", "S91_P_FCSD_HRBstp_Spd", "S91_P_FCSU_BPV_OpnCls_Time", "S91_P_FCSU_DCDC_CurrRampGrad", "S91_P_FCSU_DCDC_MaxWrmUp_Curr", "S91_P_FCSU_DCDC_OpTime", "S91_P_FCSU_DCDC_PreOpTime", "S91_P_FCSU_ETC_InitSpd", "S91_P_FCSU_GHU_StrtPress1", "S91_P_FCSU_GHU_StrtPress2", "S91_P_FCSU_H2_InitPress", "S91_P_FCSU_H2_Press_I_Ctrl", "S91_P_FCSU_H2_Press_P_Ctrl", "S91_P_FCSU_H2_StrtPress", "S91_P_FCSU_HRB_StrtSpd", "S91_P_FCSU_InitMinCellVolt", "S91_P_FCSU_MinCellVolt_Time", "S91_P_FCSU_PVrmp_IncrClsTime", "S91_P_FCSU_PVrmp_IniOpnTime", "S91_P_FCSU_PVrmp_StrtClsTime", "S91_P_FCSU_STK_DeltaMedLow_V", "S91_P_FCSU_STK_LowCellVolt", "S91_P_FCSU_STK_NormOpSet_Temp", "S91_P_HMI_BAT_SOC_Limit_low", "S91_P_HMI_BAT_SOC_Limit_ok", "S91_P_HMI_H2_leak_amb_ppm", "S91_P_HMI_H2_leak_exh_ppm", "S91_P_HMI_H2_leak_exh_s", "S91_P_HMI_H2TankLvl_Displ", "S91_P_HMI_H2TankLvl_PressLim", "S91_P_HMI_H2TankLvl_Scale0", "S91_P_HMI_H2TankLvl_Scale1", "S91_P_HRBo_a_Valve_Async_fact", "S91_P_HRBo_a_Valve_I_fact", "S91_P_HRBo_a_Valve_OT_fact", "S91_P_PC_MinUCell_range1_Time", "S91_P_PC_MinUCell_range1_Volt", "S91_P_PC_MinUCell_range2_Time", "S91_P_PC_MinUCell_range2_Volt", "S91_P_PC_UIrangeCell_Time", "S91_P_PC_UIrangeCell_Volt", "S91_P_Power_Out_FC_High", "S91_P_Power_Out_FC_Low", "S91_P_RFC_HghVent_FanSpd", "S91_P_RFC_NrmOpBaseVal_FanSpd", "S91_P_RFC_SrtStpVent_FanSpd", "S91_P_SOC_Limit_FC_High", "S91_P_SOC_Limit_FC_Low", "S91_P_SOC_Limit_FC_Off", "S91_P_SPDN_BATlimit_Curr", "S91_P_SPDN_BATlimit_Time", "S91_P_TC_ClPmpSpd_Amp0", "S91_P_TC_ClPmpSpd_Amp1", "S91_P_TC_ClPmpSpd_Amp2", "S91_P_TC_ClPmpSpd_perc0", "S91_P_TC_ClPmpSpd_perc1", "S91_P_TC_ClPmpSpd_perc2", "S91_P_TC_GHU_MaxLowPress", "S91_P_TC_GHU_MaxMidPress", "S91_P_TC_OTV_MaxTankPress", "S91_P_WTLC_SOC_Lvl", "S91_P_WTLC_SOC_time2off"}
  T3 = cluster{"Signal Name":string[], "Description":string[], "Unit":string[], "Min":dbl[], "Max":dbl[], "TestmodeA":bool[], "LogEnable":bool[]}
  T4 = cluster{"Signal Name":string[], "Description":string[], "Unit":string[], "Default":dbl[], "Min":dbl[], "Max":dbl[], "TestmodeA":bool[], "LogEnable":bool[]}
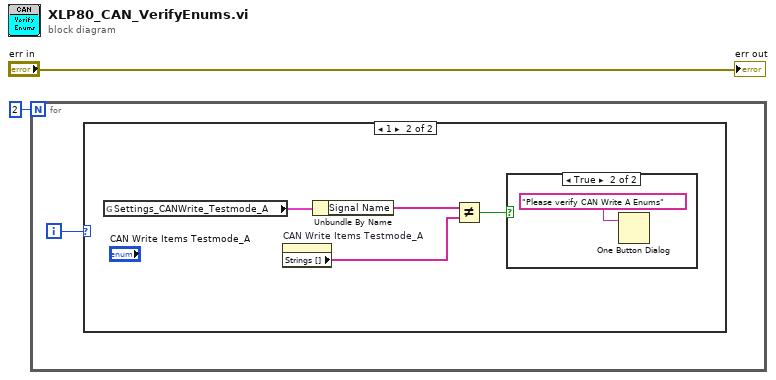
[diagram p0: block diagram]
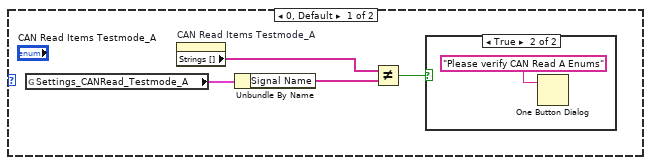
[diagram p2: hidden frame]
diagram:
  n1 = for {
    N: 2 -> [_]
    i -> [w3]
    n2 = case shown="1" w3 {
      frame 0, Default {
        n3 = global read "Globals_Settings_XLP80.vi" "Settings_CANRead_Testmode_A"() -> (w4:T3)
        n4 = property on="CAN Read Items Testmode_A" class="Enum (strict)"() -> ("Strings []"=w6:string[])  [unwired: 2 in, 2 out]
        n5 = Unbundle By Name(w4) -> ("Signal Name"=w5:string[])
        n6 = Not Equal?(x=w6, y=w5) -> (x != y?=w7:bool)
        n7 = case shown="True" w7 {
          frame False {
          }
          frame True {
            n8 = One Button Dialog(message="Please verify CAN Read A Enums") -> ()  [unwired: 1 in, 1 out]
          }
        }
      }
      frame 1 {
        n9 = global read "Globals_Settings_XLP80.vi" "Settings_CANWrite_Testmode_A"() -> (w9:T4)
        n10 = property on="CAN Write Items Testmode_A" class="Enum (strict)"() -> ("Strings []"=w11:string[])  [unwired: 2 in, 2 out]
        n11 = Unbundle By Name(w9) -> ("Signal Name"=w10:string[])
        n12 = Not Equal?(x=w10, y=w11) -> (x != y?=w12:bool)
        n13 = case shown="True" w12 {
          frame False {
          }
          frame True {
            n14 = One Button Dialog(message="Please verify CAN Write A Enums") -> ()  [unwired: 1 in, 1 out]
          }
        }
      }
    }
  }
  "err out" <- "err in"
